vi "Digitizer_5774_FPGA.vi"() -> ()   [LabVIEW 2018, in "GettingStarted_5774_FPGA.lvlib"]
uses:
  GettingStarted_5774_FPGA.lvlib
  Streaming/FIFO Utilization.ctl
  <instrlib>/_niInstr/Streaming/v1/Common/Stream State.ctl
  <vilib>/Platform/TimedLoop/XDataNode/timing_clust.ctl
  <vilib>/Platform/TimedLoop/XDataNode/nitl_modes.ctl
  <vilib>/Platform/TimedLoop/XDataNode/wakeup.ctl
  <instrlib>/FlexRIO/API/FPGA/v1/Types/Start Trigger IO Resources.ctl
  <vilib>/rvi/Emulation/niFpgaSctlEmulationGetInTimedLoop.vi
  <vilib>/rvi/Emulation/niFpgaEmulationReportErrorSimple.vi
  <vilib>/rvi/Emulation/niFpgaGetClockAttributes.vi
  <vilib>/rvi/Emulation/niFpgaCriticalErrorInLSC.vi
  <vilib>/rvi/eio/common/nirviEmuTemplateMethod_errors.vi
  <vilib>/rvi/DataTransferAndStorage/Container/Common/niFpgaContainerGetUniqueNameForEmu.vi
  <vilib>/rvi/DataTransferAndStorage/Container/Common/niFpgaContainerSetEmuInfo.vi
  <vilib>/rvi/eio/common/nirviEmuReportErrorAndStop.vi
  Streaming/SubVIs/Waveform Acquisition - Create Resources (16xI16).vi
  Streaming/SubVIs/Waveform Acquisition - Process (16xI16).vi
  2c54fa2d-4261-47aa-8496-584149bfc8f9.vi
  52314b2a-5df6-46e1-8e8c-f4aff1bd7d69.vi
  <instrlib>/_niInstr/DSP/v1/FPGA/Public/Sub VIs/Digital Offset/Digital Offset - Real - 16 spc.vi
  <instrlib>/_niInstr/DSP/v1/FPGA/Public/Sub VIs/Digital Gain/Digital Gain - Real - 16 spc.vi
  <instrlib>/_niInstr/DSP/v1/FPGA/Public/Sub VIs/HB Decimator/Halfband Decimator - IQ - 16 spc - 2x oc.vi
  <instrlib>/_niInstr/DSP/v1/FPGA/Public/Sub VIs/Fractional Decimator/Fractional Decimator - 8 spc - 2x oc.vi
  Streaming/SubVIs/Acquisition Stream Control (Real 16 SPC).vi
  Streaming/SubVIs/Waveform Acquisition - Write (16xI16).vi
  <vilib>/rvi/DataTransferAndStorage/Container/Common/niFpgaContainerExecOnDevCompGetState.vi
  <vilib>/rvi/Emulation/niFpgaEmulationIsFPGAContextNoSignature.vi
  <vilib>/rvi/Memory/Memory_Emulation/niFpgaMemoryEmulationCacheClearOnFirstRun.vi
  <vilib>/rvi/Memory/Memory_Emulation/nirvimemoryEmulationManagerCache_MakeExclusive.vi
  <vilib>/rvi/Memory/Memory_Emulation/niFpgaMemoryEmulationValidateCache.vi
  <vilib>/rvi/Memory/Memory_Emulation/nirvimemoryEmulationManagerCache_InsertValue.vi
  <vilib>/Utility/error.llb/Clear Errors.vi
  <vilib>/rvi/Memory/Memory_Emulation/nirvimemoryEmulationManagerCache_ReleaseExclusive.vi
  <vilib>/rvi/Memory/Memory_Emulation/nirvimemoryEmulationManagerCache_GetValue.vi
  <vilib>/rvi/Memory/Memory_Emulation/nirvimemoryEmulationManagerCache_SetValue.vi
  <vilib>/rvi/Emulation/niFpgaProcessEmulError.vi
  <vilib>/Platform/TimedLoop/XDataNode/XDataNode.xnode
  <vilib>/eio/EIONode/EIONode.xnode
  <vilib>/rvi/LocalResourceManager/LocalResourceManager.xnode
  <vilib>/rvi/DataTransferAndStorage/Container/XNode/niFpgaContainer.xnode
  <vilib>/rvi/DataTransferAndStorage/Register/Emulation/niFpgaRegisterEmulationRefIn.vi
  <vilib>/Platform/TimedLoop/XDataNode/XDNodeRunTimeDep.lvlib
  <instrlib>/FlexRIO/API/FPGA/v1/FlexRIO API FPGA v1.lvlib
  <instrlib>/FlexRIO/API/FPGA/v1/IO/NI5785/FlexRIO 5785 FPGA v1.lvlib
  <instrlib>/_niInstr/DSP/v1/FPGA/niInstr DSP v1 FPGA.lvlib
  <instrlib>/_niInstr/Basic Elements/v1/FPGA/niInstr Basic Elements v1 FPGA.lvlib
  Streaming/Streaming FPGA.lvlib
  <instrlib>/_niInstr/Streaming/v1/Common/niInstr Streaming v1 Common.lvlib
panel:
  in  "Tab Control":T1(tab)
  in  "trigger.monitor enable":bool
  in  "User-defined Start Trigger - AI":bool
  out "flexrio.module.io error 0":i32
  out "flexrio.module.dram ready 0":bool
  out "flexrio.module.io ready 0":bool
  out "flexrio.module.data valid 0":bool
  in  "flexrio.trigger.analog.edge.rising 0":bool=TRUE
  in  "flexrio.trigger.analog.edge.hysteresis 0":fxp<+/-,32,1>
  in  "flexrio.trigger.analog.edge.threshold 0":fxp<+/-,32,1>
  in  "flexrio.trigger.start.cfg 0":u16
  in  "flexrio.trigger.analog.edge.channel 0":fxp<+,2,2> format="%#_4g"
  in  "stream.num records 0":u64 caption="stream.num samples 0"
  out "acq.maximum delay":u16
  out "acq.wfm.memory FIFO size":u64
  out "acq.wfm.memory DRAM size":u64
  out "acq.wfm.FIFO size":u64
  in  "acq.wfm.enable bit packing 0":bool
  in  "acq.dsp.bypass":bool
  in  "flexrio.io.interleaving factor 0":u16=1
  in  "acq.dsp.delay":fxp<+/-,16,0>
  in  "acq.dsp.output sample rate":fxp<+,48,1>=1.0
  in  "acq.stream.start enable":bool
  in  "stream.initial ignore 0":u64
  in  "stream.num samples 0":u64
  in  "stream.request state 0":T2
  out "stream.state 0":T2
  out "stream.samples transferred 0":u64
  out "stream.metadata 0":u64
  in  "acq.stream.reset":bool
  out "acq.wfm.reset done":bool
  in  "acq.wfm.latch utilization":bool
  out "acq.wfm.memory utilization 0":T3
  out "acq.wfm.FIFO utilization 0":T3
  in  "acq.wfm.bypass DRAM FIFO 0":bool
  in  "acq.wfm.reset":bool
  in  "acq.dsp.integer delay":u32
  in  "acq.dsp.offset 0":fxp<+/-,18,1>
  in  "acq.dsp.gain 0":fxp<+/-,24,3>=1.0
  in  "flexrio.buffer.delay.reset 0":bool
  in  "flexrio.buffer.delay.clocks 0":u16=1
  out "flexrio.buffer.delay.ready":bool
  in  "acq.dsp.reset":bool
  out "acq.dsp.reset done":bool
  in  "acq.channels enabled":u8
  in  "acq.dsp.latch overflow":bool
  out "acq.dsp.overflow 0":bool
  out "acq.dsp.hb decimators":u8
  in  "acq.dsp.gain 1":fxp<+/-,24,3>=1.0
  in  "acq.dsp.offset 1":fxp<+/-,18,1>
  in  "acq.wfm.enable bit packing 1":bool
  in  "stream.initial ignore 1":u64
  out "stream.metadata 1":u64 caption="stream.metadata 0"
  out "stream.samples transferred 1":u64 caption="stream.samples transferred 0"
  out "stream.state 1":T2 caption="stream.state 0"
  in  "stream.request state 1":T2 caption="stream.request state 0"
  in  "stream.num samples 1":u64 caption="stream.num samples 0"
  out "acq.wfm.FIFO utilization 1":T3
  out "acq.wfm.memory utilization 1":T3
  in  "acq.wfm.bypass DRAM FIFO 1":bool
  out "acq.dsp.overflow 1":bool
  in  "stream.num records 1":u64 caption="stream.num samples 0"
  # "Trigger Configuration"
  # "Module Status"
  # "User-defined Controls"
  # "Waveform Acquisition Configuration and Status"
  # "Acquisition Stream Configuration"
  # "Acquisition DSP and Data Path Configuration"
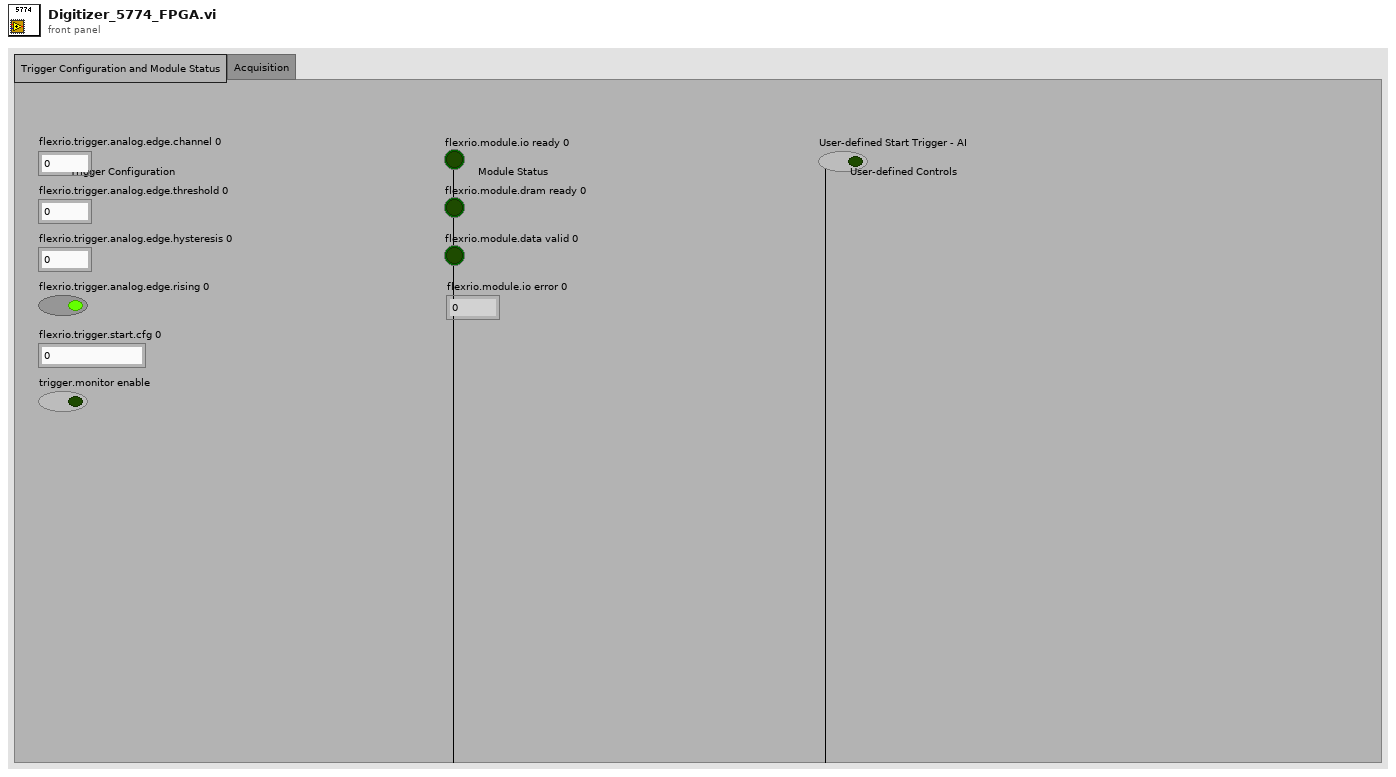
[diagram p1: front panel]
types:
  T1 = enum32{"Trigger Configuration and Module Status", "Acquisition"}
  T2 = typedef "niInstr Streaming v1 Common.lvlib/Stream State.ctl" = enum8{"Idle", "Finite Transfer", "Continuous", "Done", "Error", "Not Ready", "Cancel"}
  T3 = typedef "Streaming FPGA.lvlib/FIFO Utilization.ctl" = cluster{"lowest":u32, "highest":u32}
  T4 = typedef "Streaming FPGA.lvlib/Waveform Acquisition Resources (16xI16).ctl" = cluster{"T2H FIFO":refnum<k21>, "DRAM Clock":refnum<k21>, "DRAM Memory":refnum<k21>, "DRAM Memory Size":u32, "DRAM Ready":refnum<k21>, "Input FIFO":T5, "reset handshake item":refnum<k21>, "bypass DRAM FIFO":refnum<k21>, "read count":refnum<k21>, "elements to read":refnum<k21>}
  T5 = typedef "Streaming FPGA.lvlib/Target-Scoped FIFO (16xI16) Resource.ctl" = refnum<k21>
  T6 = typedef "XDNodeRunTimeDep.lvlib/timing_clust.ctl" = cluster{"Expected End [f-1]":u64, "Actual End [f-1]":u64, "Finished Late? [f-1]":bool, "Expected End [i-1]":u64, "Actual End [i-1]":u64, "Finished Late? [i-1]":bool, "Expected Start [i]":u64, "Actual Start [i]":u64, "Expected Start [f]":u64, "Actual Start [f]":u64, "Source Name":string, "Structure Name":string, "Period":i64, "Deadline":i64, "Offset":i64, "Start":i64, "Priority":i32, "Timeout":i32, "Mode":T7, "Wakeup Reason":T8, "Error":errorcluster, "Source Type":string, "Secondary Source Type":string, "Global End Time":u64, "Global Start Time":u64, "Frame Duration":u64, "Iteration Duration":u64, "Assigned CPU":i32, "I/O Scan Engine Mode":u32}
  T7 = typedef "XDNodeRunTimeDep.lvlib/nitl_modes.ctl" = enum32{"No Change", "Process missed periods, maintain original phase", "Discard missed periods, maintain original phase", "Process missed periods, ignore original phase", "Discard missed periods, ignore original phase"}
  T8 = typedef "XDNodeRunTimeDep.lvlib/wakeup.ctl" = enum32{"Normal", "Aborted", "Asynchronous wakeup", "Timing source error", "Timed loop error", "Timeout"}
  T9 = cluster{"flexrio.trigger.analog.edge.channel 0":fxp<+,2,2>, "flexrio.trigger.analog.edge.threshold 0":fxp<+/-,32,1>, "flexrio.trigger.analog.edge.hysteresis 0":fxp<+/-,32,1>, "flexrio.trigger.analog.edge.rising 0":bool}
  T10 = typedef "FlexRIO API FPGA v1.lvlib/Start Trigger IO Resources.ctl" = cluster{"start trigger":refnum<k21>, "started event":refnum<k21>, "start trigger for export":refnum<k21>, "start trigger for tclk":refnum<k21>}
  T11 = typedef "FlexRIO API FPGA v1.lvlib/Start Trigger Control.ctl" = cluster{"arm start":bool, "done":bool}
  T12 = typedef "niInstr DSP v1 Shared.lvlib/IQ Data.ctl" = cluster{"I":fxp<+/-,18,1>, "Q":fxp<+/-,18,1>, "overflow":bool}
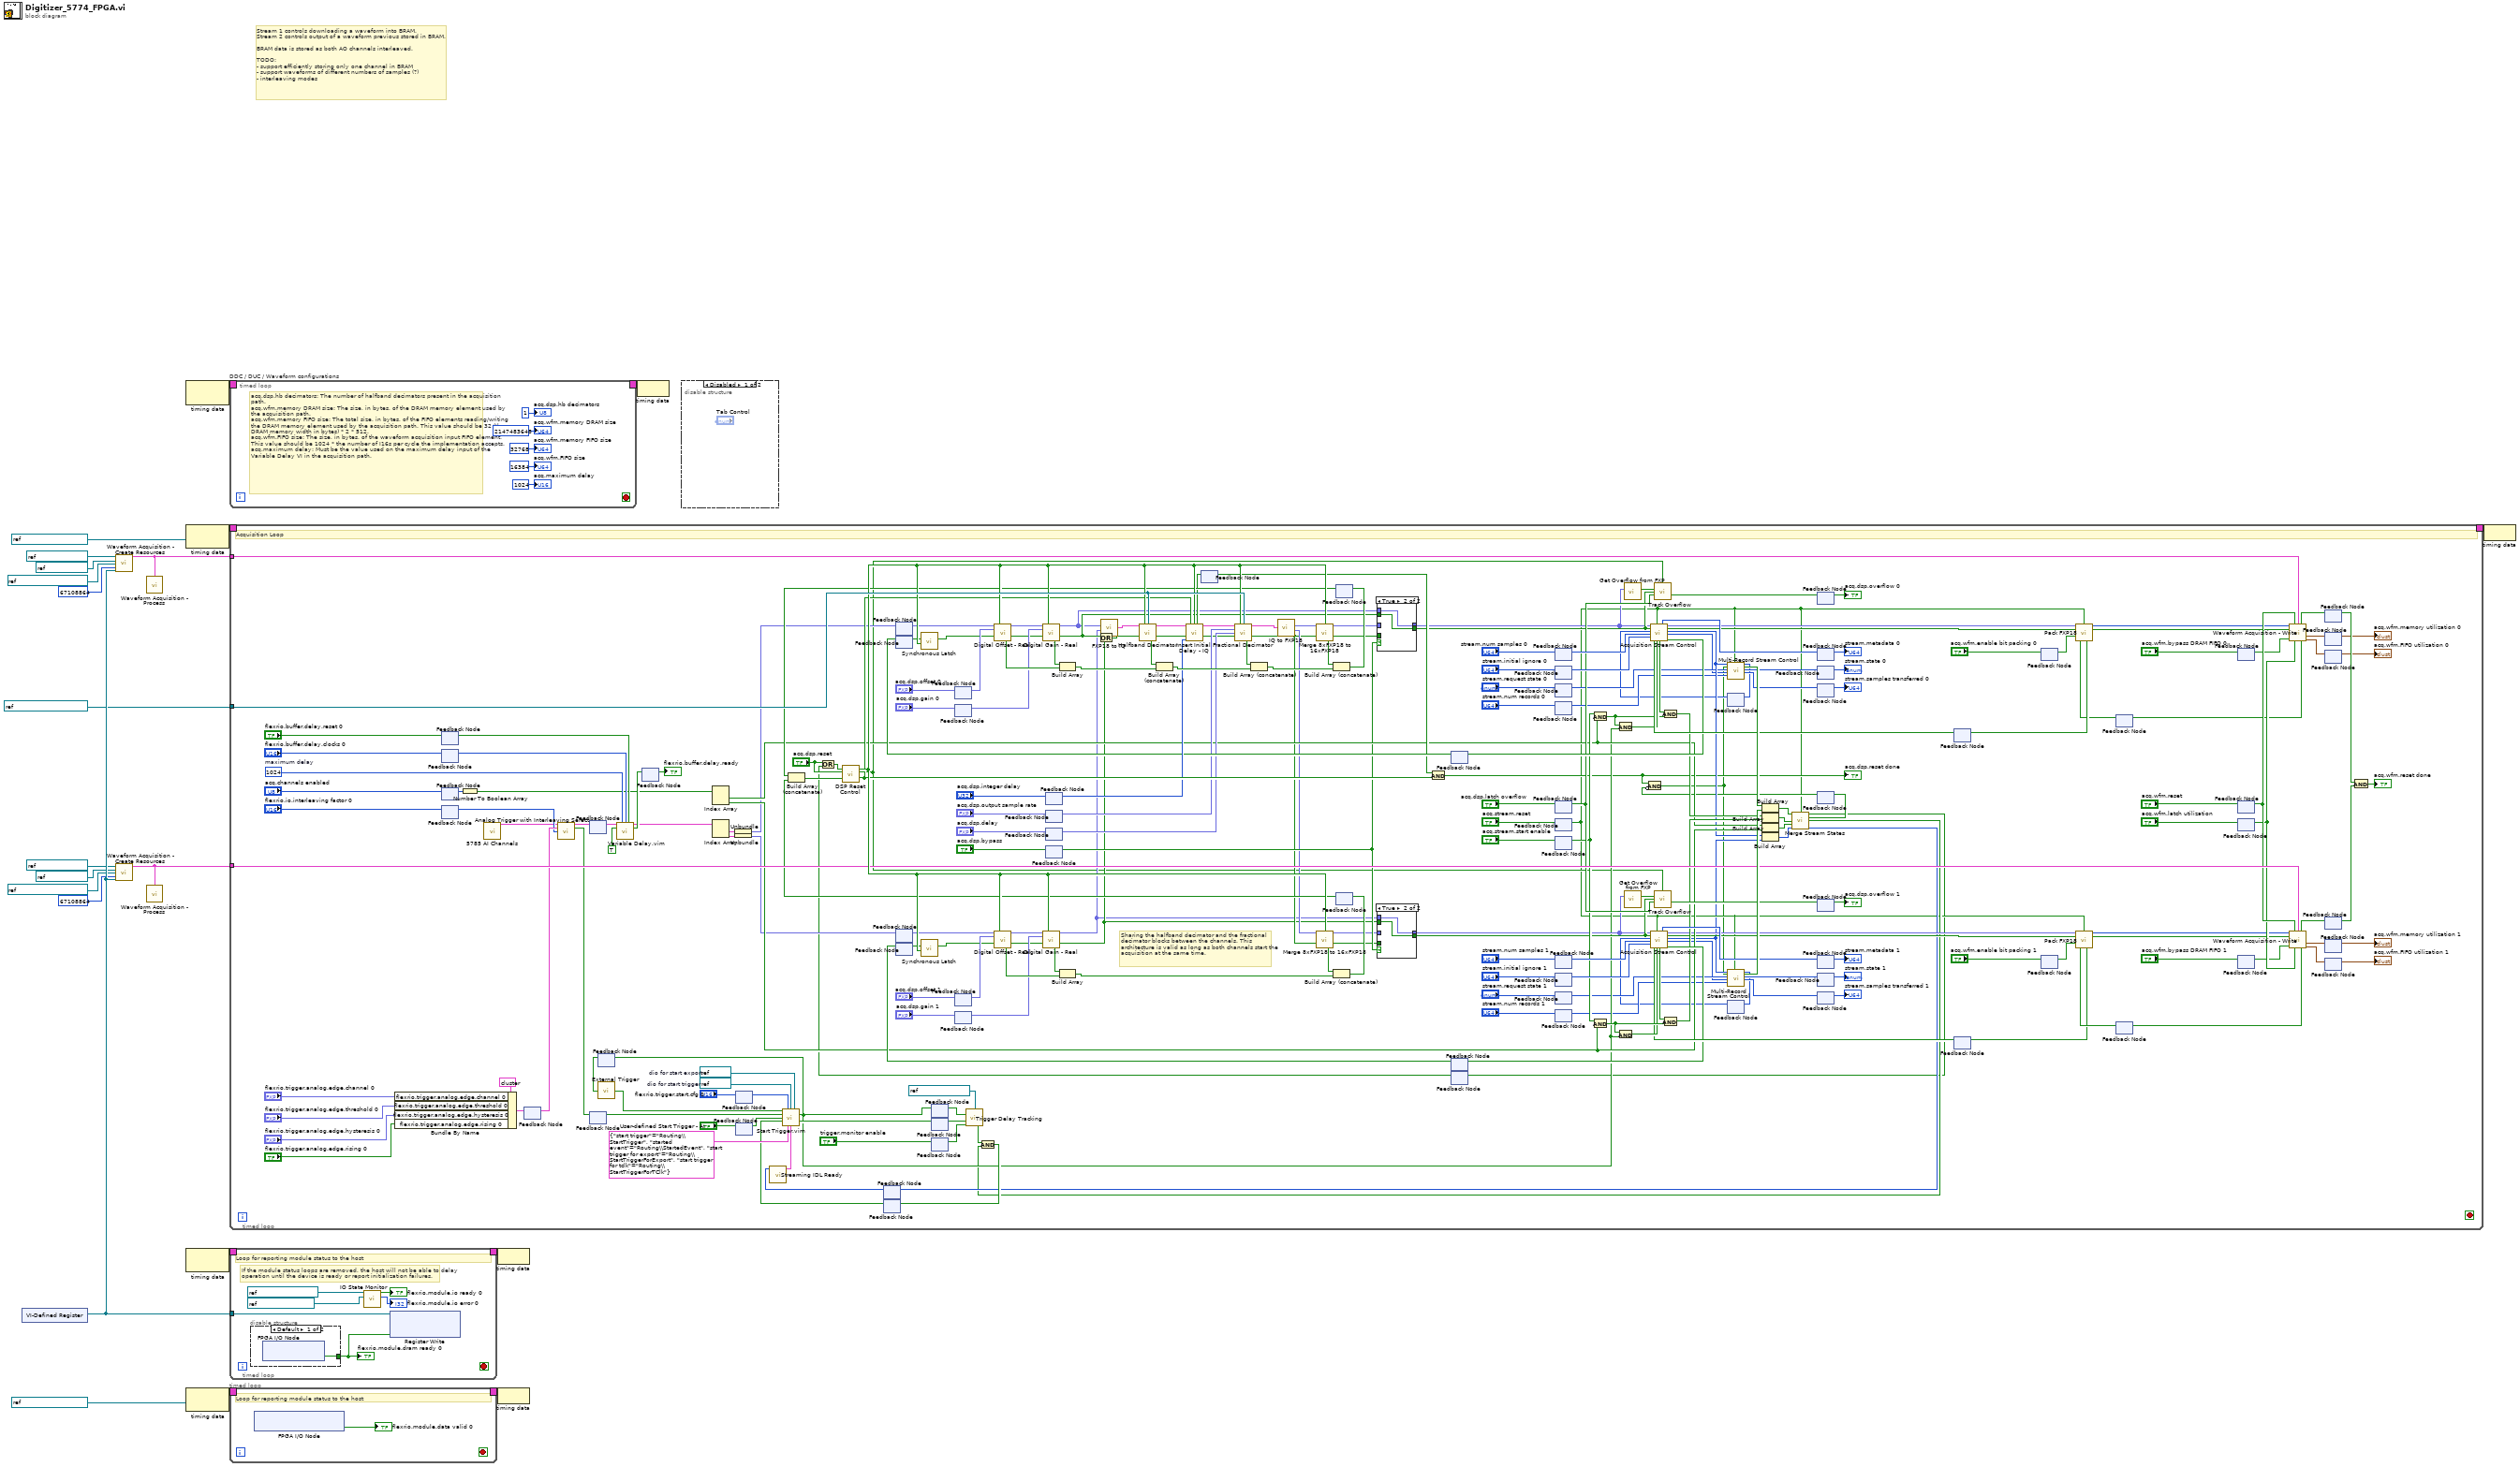
[diagram p0: block diagram]
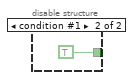
[diagram p3: hidden frame]
diagram:
  # "Stream 1 controls downloading a waveform into BRAM.\nStream 2 controls output of a waveform previous stored in BRAM.\n\nBRAM data is stored as both AO channels interleaved.\n\nTODO:\n- support efficiently storing only one channel in BRAM\n- support waveforms of different numbers of samples (?)\n- interleaving modes"
  n1 = xnode "VI-Defined Register"() -> ("Register Out"=w22:refnum<k21>)
  n2 = call-poly "Waveform Acquisition - Create Resources.vi"("T2H FIFO"=refnum<k21> "stream.to host 0", "DRAM Clock"=refnum<k21> "DRAM Clock", "DRAM Memory"=refnum<k21> "DRAM Bank0 67108864", "DRAM Memory Size"=u32 67108864 ("Memory Size"), "DRAM Ready"=w22) -> ("Waveform Acquisition Resources"=w13:T4)  [unwired: 10 in]
  n3 = call-poly "Waveform Acquisition - Create Resources.vi"("T2H FIFO"=refnum<k21> "stream.to host 1", "DRAM Clock"=refnum<k21> "DRAM Clock", "DRAM Memory"=refnum<k21> "DRAM Bank1 67108864", "DRAM Memory Size"=u32 67108864 ("Memory Size"), "DRAM Ready"=w22) -> ("Waveform Acquisition Resources"=w1:T4)  [unwired: 10 in]
  n4 = call-poly "Waveform Acquisition - Process.vi"("Waveform Acquisition Resources"=w13) -> ()  [unwired: 15 in]
  n5 = call-poly "Waveform Acquisition - Process.vi"("Waveform Acquisition Resources"=w1) -> ()  [unwired: 15 in]
  n6 = node-c288() -> (w7:T6)  [unwired: 1 in]
  n7 = node-c288(refnum<k21> "IO Socket\\Data Clock" ("Source Name")) -> (w21:T6)
  n8 = node-c288() -> (w18:T6)  [unwired: 1 in]
  n9 = node-c288(refnum<k21> "IO Socket\\Data Clock" ("Source Name")) -> (w16:T6)
  n10 = timed-loop "DDC / DUC / Waveform configurations" {
    timing: w7 -> [_]
    timing-out: [_] -> w6
    stop <- _ stop-if-true
    # "acq.dsp.hb decimators: The number of halfband decimators present in the acquisition path.\nacq.wfm.memory DRAM size: The size, in bytes, of the DRAM memory element used by the acquisition path.\nacq.wfm.memory FIFO size: The total size, in bytes, of the FIFO elements reading/writing the DRAM memory element used by the acquisition path. This value should be 32 (the DRAM memory width in bytes) * 2 * 512.\nacq.wfm.FIFO size: The size, in bytes, of the waveform acquisition input FIFO element. This value should be 1024 * the number of I16s per cycle the implementation accepts.\nacq.maximum delay: Must be the value used on the maximum delay input of the Variable Delay VI in the acquisition path."
    "acq.dsp.hb decimators" <- u8 1 ("acq.dsp.hb decimators")
    "acq.wfm.FIFO size" <- u64 16384 ("acq.wfm.FIFO size")
    "acq.wfm.memory DRAM size" <- u64 2147483648 ("acq.wfm.memory DRAM size")
    "acq.wfm.memory FIFO size" <- u64 32768 ("acq.wfm.memory FIFO size")
    "acq.maximum delay" <- u16 1024 ("acq.maximum delay")
  }
  n11 = timed-loop {
    timing: w21 -> [_]
    timing-out: [_] -> w20
    tunnel: refnum<k21> "IO Socket\\Data Clock 2x" ("Source Name") -> [w270]
    tunnel: w13 -> [w268]
    tunnel: w1 -> [w267]
    stop <- _ stop-if-true
    w242 = u16 1024  # maximum delay
    w246 = refnum<k21> "DIO 0"  # dio for start trigger
    w245 = refnum<k21> "DIO 1"  # dio for start export
    # "Sharing the halfband decimator and the fractional decimator blocks between the channels. This architecture is valid as long as both channels start the acquisition at the same time."
    # "Acquisition Loop"
    n12 = Bundle By Name(cluster=T9 {"flexrio.trigger.analog.edge.channel 0"=0.0, "flexrio.trigger.analog.edge.threshold 0"=0.0, "flexrio.trigger.analog.edge.hysteresis 0"=0.0, "flexrio.trigger.analog.edge.rising 0"=FALSE} ("config"), "flexrio.trigger.analog.edge.channel 0"="flexrio.trigger.analog.edge.channel 0", "flexrio.trigger.analog.edge.threshold 0"="flexrio.trigger.analog.edge.threshold 0", "flexrio.trigger.analog.edge.hysteresis 0"="flexrio.trigger.analog.edge.hysteresis 0", "flexrio.trigger.analog.edge.rising 0"="flexrio.trigger.analog.edge.rising 0") -> (w227:T9)
    n13 = feedback #1() -> (w224:bool)  [unwired: 1 in]
    n14 = feedback-in #1("flexrio.buffer.delay.reset 0") -> ()
    n15 = feedback #2() -> (w222:u16)  [unwired: 1 in]
    n16 = feedback-in #2("flexrio.buffer.delay.clocks 0") -> ()
    n17 = feedback #3() -> (w181:u8)  [unwired: 1 in]
    n18 = feedback-in #3("acq.channels enabled") -> ()
    n19 = feedback #4() -> (w186:u16)  [unwired: 1 in]
    n20 = feedback-in #4("flexrio.io.interleaving factor 0") -> ()
    n21 = Number To Boolean Array(number=w181) -> (Boolean array=w180:bool[])
    n22 = call <instrlib>:"5785 AI Channels.vi"() -> ("all channels"=w101:cluster{fxp<+/-,12,1>[]}[])  [unwired: 15 in]
    n23 = feedback-in #5(w227) -> ()
    n24 = feedback #5() -> (w191:T9)  [unwired: 1 in]
    n25 = call "Analog Trigger with Interleaving Select.vi"("all channels"=w101, "config"=w191, "interleaving factor"=w186) -> ("all channels delayed out"=w99:cluster{fxp<+/-,12,1>[]}[], "triggered"=w241:bool)  [unwired: 11 in]
    n26 = feedback #6() -> (w100:cluster{fxp<+/-,12,1>[]}[])  [unwired: 1 in]
    n27 = feedback-in #6(w99) -> ()
    n28 = feedback-in #7(w241) -> ()
    n29 = feedback #7() -> (w232:bool)  [unwired: 1 in]
    n30 = feedback #8() -> (w90:bool)  [unwired: 1 in]
    n31 = call "External Trigger.vi"("front panel trigger out"=w90) -> ("front panel trigger in"=w89:bool)  [unwired: 4 in]
    n32 = call "Variable Delay.vim"("Array in"=w100, "maximum delay"=w242, "delay"=w222, "reset"=w224, "data valid"=TRUE) -> ("Array out"=w98:cluster{fxp<+/-,12,1>[]}[], "data valid?"=w197:bool)  [unwired: 8 in, 1 out]
    n33 = feedback-in #9(w197) -> ()
    n34 = feedback #9() -> (→"flexrio.buffer.delay.ready":bool)  [unwired: 1 in]
    n35 = Index Array(array=w180) -> (element #1=w123:bool, element #2=w122:bool)  [unwired: 2 in]
    n36 = Index Array(array=w98) -> (element #1=w185:cluster{fxp<+/-,12,1>[]}, element #2=w184:cluster{fxp<+/-,12,1>[]})  [unwired: 2 in]
    n37 = Unbundle(w185) -> (w103:fxp<+/-,12,1>[])
    n38 = Unbundle(w184) -> (w102:fxp<+/-,12,1>[])
    n39 = feedback-in #10("flexrio.trigger.start.cfg 0") -> ()
    n40 = feedback #10() -> (w194:u16)  [unwired: 1 in]
    n41 = feedback #11() -> (w192:bool)  [unwired: 1 in]
    n42 = feedback-in #11("User-defined Start Trigger - AI") -> ()
    n43 = feedback #12() -> (w244:T2)  [unwired: 1 in]
    n44 = call <instrlib>:"Streaming IDL Ready.vi"("stream.state"=w244) -> ("start trigger control"=w247:T11)  [unwired: 10 in]
    n45 = feedback #13() -> (w236:bool)  [unwired: 1 in]
    n46 = call "Start Trigger.vim"("external analog trigger"=w89, "flexrio.trigger.start.cfg 0"=w194, "dio start"=w246, "dio for start export"=w245, "analog trigger"=w232, "user-defined start trigger"=w192, "ready for start?"=w236, "trigger io resources"=T10 {"start trigger"="Routing\\StartTrigger", "started event"="Routing\\StartedEvent", "start trigger for export"="Routing\\StartTriggerForExport", "start trigger for tclk"="Routing\\StartTriggerForTClk"}, "start trigger control"=w247) -> ("conditioned start trigger"=w65:bool, "unconditioned start trigger"=w67:bool)  [unwired: 4 in, 1 out]
    n47 = feedback-in #8(w65) -> ()
    n48 = feedback #14() -> (w75:fxp<+/-,12,1>[])  [unwired: 1 in]
    n49 = feedback-in #14(w103) -> ()
    n50 = feedback #15() -> (w182:bool)  [unwired: 1 in]
    n51 = feedback #16() -> (w72:fxp<+/-,12,1>[])  [unwired: 1 in]
    n52 = feedback-in #16(w102) -> ()
    n53 = feedback #17() -> (w161:bool)  [unwired: 1 in]
    n54 = feedback #18() -> (w64:bool)  [unwired: 1 in]
    n55 = feedback-in #18(w65) -> ()
    n56 = feedback #19() -> (w66:bool)  [unwired: 1 in]
    n57 = feedback-in #19(w67) -> ()
    n58 = feedback-in #20("trigger.monitor enable") -> ()
    n59 = feedback #20() -> (w96:bool)  [unwired: 1 in]
    n60 = feedback-in #21("acq.dsp.offset 0") -> ()
    n61 = feedback #21() -> (w178:fxp<+/-,18,1>)  [unwired: 1 in]
    n62 = feedback #22() -> (w176:fxp<+/-,24,3>)  [unwired: 1 in]
    n63 = feedback-in #22("acq.dsp.gain 0") -> ()
    n64 = feedback #23() -> (w163:fxp<+/-,18,1>)  [unwired: 1 in]
    n65 = feedback-in #23("acq.dsp.offset 1") -> ()
    n66 = feedback #24() -> (w165:fxp<+/-,24,3>)  [unwired: 1 in]
    n67 = feedback-in #24("acq.dsp.gain 1") -> ()
    n68 = call "Trigger Delay Tracking.vi"("Delay Data FIFO"=refnum<k21> "trigger.to host 0", "conditioned start trigger"=w64, "unconditioned start trigger"=w66, "enable"=w96) -> ("ready for input"=w95:bool)  [unwired: 11 in]
    n69 = feedback #25() -> (w189:u32)  [unwired: 1 in]
    n70 = feedback-in #25("acq.dsp.integer delay") -> ()
    n71 = feedback #26() -> (w175:fxp<+,48,1>)  [unwired: 1 in]
    n72 = feedback-in #26("acq.dsp.output sample rate") -> ()
    n73 = feedback #27() -> (w174:fxp<+/-,16,0>)  [unwired: 1 in]
    n74 = feedback-in #27("acq.dsp.delay") -> ()
    n75 = feedback-in #28("acq.dsp.bypass") -> ()
    n76 = feedback #28() -> (w88:bool)  [unwired: 1 in]
    n77 = feedback #29() -> (w126:bool)  [unwired: 1 in]
    n78 = feedback #30() -> (w254:bool[])  [unwired: 1 in]
    n79 = feedback #31() -> (w253:bool[])  [unwired: 1 in]
    n80 = Build Array (concatenate)(w254, w253) -> (w159:bool[])
    n81 = feedback #32() -> (w183:bool)  [unwired: 1 in]
    n82 = feedback-in #15(w183) -> ()
    n83 = feedback #33() -> (w160:bool)  [unwired: 1 in]
    n84 = feedback-in #17(w160) -> ()
    n85 = feedback #34() -> (w30:bool)  [unwired: 1 in]
    n86 = Or(x="acq.dsp.reset", y=w30) -> (x .or. y?=w57:bool)
    n87 = call "DSP Reset Control.vi"("reset in"=w57, "mask 1"="acq.dsp.reset", "ready for input"=w159) -> ("reset out"=w269:bool, "masked 1 reset out"=w56:bool, "reset done"=w252:bool)  [unwired: 13 in, 1 out]
    n88 = call <instrlib>:"Synchronous Latch.vi"("clear"=w269, "set"=w182) -> ("out"=w74:bool)  [unwired: 9 in]
    n89 = call <instrlib>:"Synchronous Latch.vi"("clear"=w269, "set"=w161) -> ("out"=w71:bool)  [unwired: 9 in]
    n90 = call-poly <instrlib>:"Digital Offset - Real.vi"("data in"=w75, "reset"=w269, "offset"=w178, "input valid"=w74) -> ("data out"=w109:fxp<+/-,18,1>[], "output valid"=w108:bool, "ready for input"=w262:bool)  [unwired: 8 in, 1 out]
    n91 = call-poly <instrlib>:"Digital Offset - Real.vi"("data in"=w72, "reset"=w269, "offset"=w163, "input valid"=w71) -> ("data out"=w110:fxp<+/-,18,1>[], "output valid"=w111:bool, "ready for input"=w264:bool)  [unwired: 8 in, 1 out]
    n92 = call-poly <instrlib>:"Digital Gain - Real.vi"("data in"=w109, "reset"=w269, "gain"=w176, "input valid"=w108) -> ("data out"=w68:fxp<+/-,18,1>[], "output valid"=w73:bool, "ready for input"=w261:bool)  [unwired: 8 in, 1 out]
    n93 = call-poly <instrlib>:"Digital Gain - Real.vi"("data in"=w110, "reset"=w269, "gain"=w165, "input valid"=w111) -> ("data out"=w69:fxp<+/-,18,1>[], "output valid"=w70:bool, "ready for input"=w265:bool)  [unwired: 8 in, 1 out]
    n94 = Build Array(w261, w262) -> (w259:bool[])
    n95 = Build Array(w265, w264) -> (w79:bool[])
    n96 = Or(x=w73, y=w70) -> (x .or. y?=w76:bool)
    n97 = call "FXP18 to IQ.vi"("I in"=w68, "Q in"=w69) -> ("data out"=w84:T12[])  [unwired: 6 in]
    n98 = call-poly <instrlib>:"Halfband Decimator.vi"("data in"=w84, "reset"=w269, "clock x 2"=w270, "input valid"=w76) -> ("data out"=w85:T12[], "output valid"=w107:bool, "ready for input"=w260:bool)  [unwired: 8 in, 1 out]
    n99 = Build Array (concatenate)(w260, w259) -> (w257:bool[])
    n100 = call "Insert Initial Delay - IQ.vi"("data in"=w85, "insert"=w252, "reset"=w269, "input valid"=w107, "delay"=w189) -> ("done"=w188:bool, "data out"=w106:T12[], "output valid"=w105:bool)  [unwired: 8 in]
    n101 = feedback-in #29(w188) -> ()
    n102 = call-poly <instrlib>:"Fractional Decimator.vi"("data in"=w106, "reset"=w269, "clock x 2"=w270, "output sample rate"=w175, "delay"=w174, "input valid"=w105) -> ("data out"=w104:T12[], "output valid"=w77:bool, "ready for input"=w258:bool)  [unwired: 6 in, 1 out]
    n103 = Build Array (concatenate)(w258, w257) -> (w80:bool[])
    n104 = call "IQ to FXP18.vi"("data in"=w104) -> ("I out"=w81:fxp<+/-,18,1>[], "Q out"=w78:fxp<+/-,18,1>[])  [unwired: 8 in]
    n105 = call "Merge 8xFXP18 to 16xFXP18.vi"("data in"=w81, "reset"=w269, "input valid"=w77) -> ("data out"=w83:fxp<+/-,18,1>[], "output valid"=w82:bool, "ready for input"=w256:bool)  [unwired: 10 in]
    n106 = call "Merge 8xFXP18 to 16xFXP18.vi"("data in"=w78, "reset"=w269, "input valid"=w77) -> ("data out"=w86:fxp<+/-,18,1>[], "output valid"=w87:bool, "ready for input"=w266:bool)  [unwired: 10 in]
    n107 = Build Array (concatenate)(w256, w80) -> (w255:bool[])
    n108 = Build Array (concatenate)(w266, w79) -> (w263:bool[])
    n109 = feedback-in #30(w255) -> ()
    n110 = feedback-in #31(w263) -> ()
    n111 = case shown="True" w88 {
      tunnel: w68 -> [_ w280]
      tunnel: [w278 w280] -> w113
      tunnel: w83 -> [w278 _]
      tunnel: [w277 w279] -> w115
      tunnel: w82 -> [w277 _]
      tunnel: w73 -> [_ w279]
      frame False {
      }
      frame True {
      }
    }
    n112 = case shown="True" w88 {
      tunnel: w69 -> [_ w276]
      tunnel: [w274 w276] -> w112
      tunnel: w86 -> [w274 _]
      tunnel: [w273 w275] -> w114
      tunnel: w87 -> [w273 _]
      tunnel: w70 -> [_ w275]
      frame False {
      }
      frame True {
      }
    }
    n113 = Compound Arithmetic op=AND(w126, w252) -> (w43:bool)
    "acq.dsp.reset done" <- w43
    n114 = feedback #35() -> (w205:u64)  [unwired: 1 in]
    n115 = feedback-in #35("stream.num samples 0") -> ()
    n116 = feedback #36() -> (w203:u64)  [unwired: 1 in]
    n117 = feedback-in #36("stream.initial ignore 0") -> ()
    n118 = feedback #37() -> (w50:T2)  [unwired: 1 in]
    n119 = feedback-in #37("stream.request state 0") -> ()
    n120 = feedback #38() -> (w47:u64)  [unwired: 1 in]
    n121 = feedback-in #38("stream.num records 0") -> ()
    n122 = feedback-in #39("acq.dsp.latch overflow") -> ()
    n123 = feedback #39() -> (w129:bool)  [unwired: 1 in]
    n124 = feedback #40() -> (w41:bool)  [unwired: 1 in]
    n125 = feedback-in #40("acq.stream.reset") -> ()
    n126 = feedback #41() -> (w128:bool)  [unwired: 1 in]
    n127 = feedback-in #41("acq.stream.start enable") -> ()
    n128 = feedback #42() -> (w145:u64)  [unwired: 1 in]
    n129 = feedback-in #42("stream.num samples 1") -> ()
    n130 = feedback #43() -> (w147:u64)  [unwired: 1 in]
    n131 = feedback-in #43("stream.initial ignore 1") -> ()
    n132 = feedback #44() -> (w37:T2)  [unwired: 1 in]
    n133 = feedback-in #44("stream.request state 1") -> ()
    n134 = feedback #45() -> (w36:u64)  [unwired: 1 in]
    n135 = feedback-in #45("stream.num records 1") -> ()
    n136 = And(x=w128, y=w123) -> (x .and. y?=w166:bool)
    n137 = And(x=w128, y=w122) -> (x .and. y?=w158:bool)
    n138 = And(x=w166, y=w65) -> (x .and. y?=w238:bool)
    n139 = And(x=w158, y=w65) -> (x .and. y?=w132:bool)
    n140 = call "Get Overflow from FXP.vi"("data in"=w113) -> ("overflow out"=w173:bool[])  [unwired: 14 in]
    n141 = call "Get Overflow from FXP.vi"("data in"=w112) -> ("overflow out"=w152:bool[])  [unwired: 14 in]
    n142 = call "Track Overflow.vi"("reset"=w56, "overflow in"=w173, "input valid"=w115, "latch overflow status"=w129) -> ("overflow detected"=w210:bool)  [unwired: 11 in]
    n143 = call "Track Overflow.vi"("reset"=w56, "overflow in"=w152, "input valid"=w114, "latch overflow status"=w129) -> ("overflow detected"=w141:bool)  [unwired: 11 in]
    n144 = feedback #46() -> (w45:T2)  [unwired: 1 in]
    n145 = feedback #47() -> (w32:T2)  [unwired: 1 in]
    n146 = Build Array(w123, w122) -> (w60:bool[])
    n147 = feedback #48() -> (→"acq.dsp.overflow 0":bool)  [unwired: 1 in]
    n148 = feedback-in #48(w210) -> ()
    n149 = feedback #49() -> (→"stream.metadata 0":u64)  [unwired: 1 in]
    n150 = feedback #50() -> (→"stream.state 0":T2)  [unwired: 1 in]
    n151 = feedback #51() -> (→"stream.samples transferred 0":u64)  [unwired: 1 in]
    n152 = feedback #52() -> (w42:bool)  [unwired: 1 in]
    n153 = Compound Arithmetic op=AND(w43, invert w42) -> (w38:bool)
    n154 = feedback #53() -> (→"acq.dsp.overflow 1":bool)  [unwired: 1 in]
    n155 = feedback-in #53(w141) -> ()
    n156 = feedback #54() -> (→"stream.metadata 1":u64)  [unwired: 1 in]
    n157 = feedback #55() -> (→"stream.state 1":T2)  [unwired: 1 in]
    n158 = feedback #56() -> (→"stream.samples transferred 1":u64)  [unwired: 1 in]
    n159 = feedback #57() -> (w239:bool)  [unwired: 1 in]
    n160 = call-poly "Acquisition Stream Control.vi"("data in"=w113, "input valid"=w115, "request state"=w45, "num samples"=w205, "initial ignore"=w203, "ready for output (T)"=w239, "reset"=w41, "start trigger"=w238) -> ("ready for start"=w237:bool, "metadata"=w199:u64, "data out"=w117:fxp<+/-,18,1>[], "output valid"=w116:bool, "actual state"=w53:T2, "samples transferred"=w49:u64, "acquiring"=w235:bool)  [unwired: 5 in]
    n161 = feedback-in #32(w235) -> ()
    n162 = And(x=w237, y=w166) -> (x .and. y?=w125:bool)
    n163 = call "Multi-Record Stream Control.vi"("actual state from slave"=w53, "ready to restart"=w38, "request state"=w50, "samples transferred"=w49, "num records"=w47, "reset"=w41) -> ("request state to slave"=w46:T2, "request to restart"=w272:bool, "actual state"=w52:T2, "total samples transferred"=w48:u64)  [unwired: 10 in]
    n164 = feedback-in #46(w46) -> ()
    n165 = feedback-in #49(w199) -> ()
    n166 = feedback-in #50(w52) -> ()
    n167 = feedback-in #51(w48) -> ()
    n168 = feedback #58() -> (w131:bool)  [unwired: 1 in]
    n169 = call-poly "Acquisition Stream Control.vi"("data in"=w112, "input valid"=w114, "request state"=w32, "num samples"=w145, "initial ignore"=w147, "ready for output (T)"=w131, "reset"=w41, "start trigger"=w132) -> ("ready for start"=w133:bool, "metadata"=w150:u64, "data out"=w91:fxp<+/-,18,1>[], "output valid"=w92:bool, "actual state"=w39:T2, "samples transferred"=w35:u64, "acquiring"=w130:bool)  [unwired: 5 in]
    n170 = feedback-in #33(w130) -> ()
    n171 = And(x=w133, y=w158) -> (x .and. y?=w124:bool)
    n172 = call "Multi-Record Stream Control.vi"("actual state from slave"=w39, "ready to restart"=w38, "request state"=w37, "samples transferred"=w35, "num records"=w36, "reset"=w41) -> ("request state to slave"=w33:T2, "request to restart"=w271:bool, "actual state"=w40:T2, "total samples transferred"=w34:u64)  [unwired: 10 in]
    n173 = feedback-in #47(w33) -> ()
    n174 = Build Array(w272, w271) -> (w51:bool[])
    n175 = Build Array(w125, w124) -> (w59:bool[])
    n176 = Build Array(w53, w39) -> (w61:T2[])
    n177 = call "Merge Stream States.vi"("request to restart"=w51, "reset"=w41, "ready for start in"=w59, "enable"=w60, "state in"=w61) -> ("request to restart out"=w31:bool, "ready to restart disable"=w44:bool, "ready for start out"=w62:bool, "state out"=w63:T2)  [unwired: 7 in]
    n178 = feedback-in #12(w63) -> ()
    n179 = And(x=w95, y=w62) -> (x .and. y?=w94:bool)
    n180 = feedback-in #13(w94) -> ()
    n181 = feedback-in #34(w31) -> ()
    n182 = feedback-in #52(w44) -> ()
    n183 = feedback-in #54(w150) -> ()
    n184 = feedback-in #55(w40) -> ()
    n185 = feedback-in #56(w34) -> ()
    n186 = feedback-in #59("acq.wfm.enable bit packing 0") -> ()
    n187 = feedback #59() -> (w169:bool)  [unwired: 1 in]
    n188 = feedback #60() -> (w155:bool)  [unwired: 1 in]
    n189 = feedback-in #60("acq.wfm.enable bit packing 1") -> ()
    n190 = feedback #61() -> (w167:bool)  [unwired: 1 in]
    n191 = call "Pack FXP18.vi"("data in"=w117, "reset"=w41, "input valid"=w116, "enable bit packing? (T)"=w169, "ready for output (T)"=w167) -> ("data out"=w121:i16[], "output valid"=w120:bool, "ready for input"=w168:bool)  [unwired: 8 in]
    n192 = feedback-in #57(w168) -> ()
    n193 = feedback #62() -> (w157:bool)  [unwired: 1 in]
    n194 = call "Pack FXP18.vi"("data in"=w91, "reset"=w41, "input valid"=w92, "enable bit packing? (T)"=w155, "ready for output (T)"=w157) -> ("data out"=w118:i16[], "output valid"=w119:bool, "ready for input"=w156:bool)  [unwired: 8 in]
    n195 = feedback-in #58(w156) -> ()
    n196 = feedback #63() -> (w217:bool)  [unwired: 1 in]
    n197 = feedback-in #63("acq.wfm.bypass DRAM FIFO 0") -> ()
    n198 = feedback-in #64("acq.wfm.reset") -> ()
    n199 = feedback #64() -> (w251:bool)  [unwired: 1 in]
    n200 = feedback #65() -> (w250:bool)  [unwired: 1 in]
    n201 = feedback-in #65("acq.wfm.latch utilization") -> ()
    n202 = feedback #66() -> (w135:bool)  [unwired: 1 in]
    n203 = feedback-in #66("acq.wfm.bypass DRAM FIFO 1") -> ()
    n204 = call-poly "Waveform Acquisition - Write.vi"("data in"=w121, "reset"=w251, "Waveform Acquisition Resources"=w268, "input valid"=w120, "bypass DRAM FIFO (F)"=w217, "latch utilization"=w250) -> ("reset done"=w216:bool, "memory utilization"=w215:T3, "ready for input"=w171:bool, "FIFO utilization"=w213:T3)  [unwired: 6 in]
    n205 = feedback-in #61(w171) -> ()
    n206 = call-poly "Waveform Acquisition - Write.vi"("data in"=w118, "reset"=w251, "Waveform Acquisition Resources"=w267, "input valid"=w119, "bypass DRAM FIFO (F)"=w135, "latch utilization"=w250) -> ("reset done"=w136:bool, "memory utilization"=w137:T3, "ready for input"=w153:bool, "FIFO utilization"=w139:T3)  [unwired: 6 in]
    n207 = feedback-in #62(w153) -> ()
    n208 = feedback #67() -> (w248:bool)  [unwired: 1 in]
    n209 = feedback-in #67(w216) -> ()
    n210 = feedback #68() -> (→"acq.wfm.memory utilization 0":T3)  [unwired: 1 in]
    n211 = feedback-in #68(w215) -> ()
    n212 = feedback #69() -> (→"acq.wfm.FIFO utilization 0":T3)  [unwired: 1 in]
    n213 = feedback-in #69(w213) -> ()
    n214 = feedback #70() -> (w249:bool)  [unwired: 1 in]
    n215 = feedback-in #70(w136) -> ()
    n216 = feedback #71() -> (→"acq.wfm.memory utilization 1":T3)  [unwired: 1 in]
    n217 = feedback-in #71(w137) -> ()
    n218 = feedback #72() -> (→"acq.wfm.FIFO utilization 1":T3)  [unwired: 1 in]
    n219 = feedback-in #72(w139) -> ()
    n220 = And(x=w248, y=w249) -> (x .and. y?=→"acq.wfm.reset done":bool)
  }
  n221 = timed-loop {
    timing: w18 -> [_]
    timing-out: [_] -> w17
    tunnel: w22 -> [w284]
    stop <- _ stop-if-true
    # "If the module status loops are removed, the host will not be able to delay operation until the device is ready or report initialization failures."
    # "Loop for reporting module status to the host"
    n222 = disable-structure shown="Default" {
      disable-tunnel: [w289 TRUE ("flexrio.module.dram ready 0")] -> w283
      frame condition #0 (active) {
        n223 = xnode "FPGA I/O Node"() -> ("DRAM Ready"=w289:bool)  [unwired: 1 in, 1 out]
      }
      frame condition #1 {
      }
    }
    "flexrio.module.dram ready 0" <- w283
    n224 = call <instrlib>:"IO State Monitor.vi"("io error resource"=refnum<k21> "IO Socket\\IO Error" ("FPGA I/O In"), "io ready resource"=refnum<k21> "IO Socket\\IO Ready" ("FPGA I/O In")) -> ("flexrio.module.io error 0"=→"flexrio.module.io error 0":i32, "flexrio.module.io ready 0"=→"flexrio.module.io ready 0":bool)  [unwired: 8 in]
    n225 = xnode ("Register Write")("Data"=w283, "Register In"=w284) -> ()  [unwired: 1 out]
  }
  n226 = timed-loop {
    timing: w16 -> [_]
    timing-out: [_] -> w15
    stop <- _ stop-if-true
    # "Loop for reporting module status to the host"
    n227 = xnode "FPGA I/O Node"() -> ("IO Socket\\AI Data Valid"=→"flexrio.module.data valid 0":bool)  [unwired: 1 in, 1 out]
  }
  n228 = node-c288(w17) -> ()
  n229 = node-c288(w15) -> ()
  n230 = node-c288(w6) -> ()
  n231 = disable-structure shown="Disabled" {
    frame Disabled {
    }
    frame Enabled {
    }
  }
  n232 = node-c288(w20) -> ()
